vi "LV SciSDK CUSTOM PACKET MULTIPLE.vi"(5 "Buffer Size":u32=1, 7 "CP Handle In":cluster{"CP Path":string, "CP Name":string}, 9 "Handle In":T1, 11 "error in (no error)":errorcluster) -> (4 "NI Error Code":i32, 6 "CP Buffer Out":T2, 8 "CP Handle Out":cluster{"CP Path":string, "CP Name":string}, 10 "Handle Out":T1, 15 "error out":errorcluster)   [LabVIEW 2021, in "SciSDK_Labview.lvlib"]
doc: "You need this VI to read multiple custom packets."
uses:
  SciSDK_Labview.lvlib
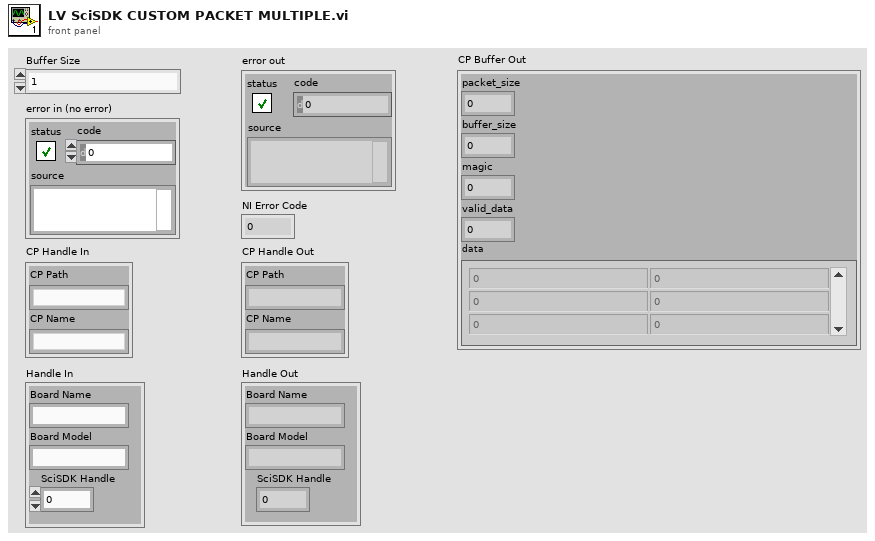
[diagram p1: front panel]
types:
  T1 = cluster{"Board Name":string, "Board Model":string, "SciSDK Handle":u64}
  T2 = cluster{"packet_size":u32, "buffer_size":u32, "magic":u32, "valid_data":dbl, "data":u32[][]}
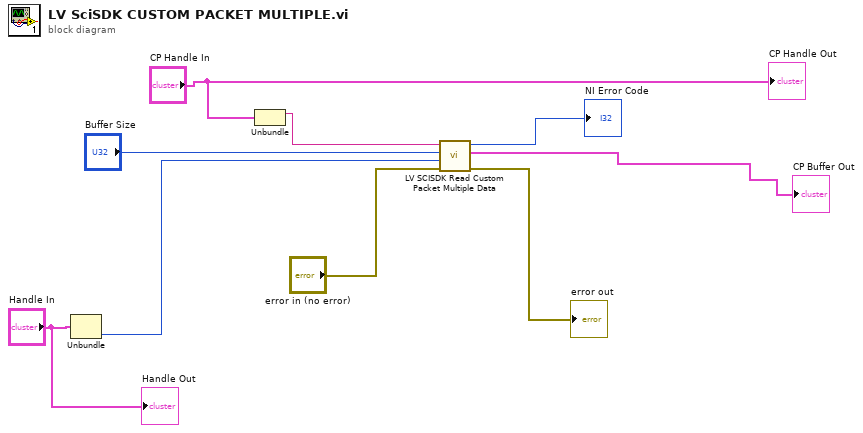
[diagram p0: block diagram]
diagram:
  n1 = Unbundle("Handle In") -> ("SciSDK Handle"=w2:u64)  [unwired: 2 out]
  n2 = Unbundle("CP Handle In") -> ("CP Path"=w3:string)  [unwired: 1 out]
  n3 = call "LV SCISDK Read Custom Packet Multiple Data.vi"("Path"=w3, "buffer size"="Buffer Size", "handle"=w2, "error in (no error)"="error in (no error)") -> ("function return"=→"NI Error Code":i32, "buffer out"=→"CP Buffer Out":T2, "error out"=→"error out":errorcluster)  [unwired: 3 in, 1 out]
  "CP Handle Out" <- "CP Handle In"
  "Handle Out" <- "Handle In"
